vi "SR201_set_state2.vi"(8 "error in":errorcluster, 9 "state_ch2":bool, 10 "state_ch1":bool, 11 "conn_id_in":refnum<k5>) -> (0 "error out":errorcluster, 1 "ch2":bool, 2 "ch1":bool, 3 "conn_id_out":refnum<k5>, 4 "status":bool, 5 "string":string)   [LabVIEW 2019]
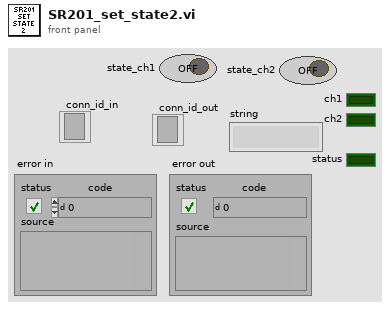
[diagram p1: front panel]
types:
  T1 = enum16{"Standard", "Buffered", "CRLF", "Immediate"}
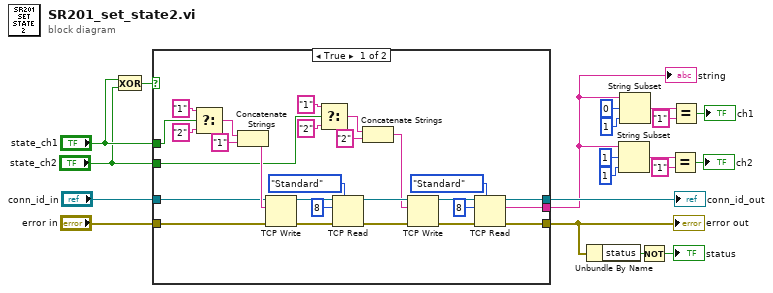
[diagram p0: block diagram]
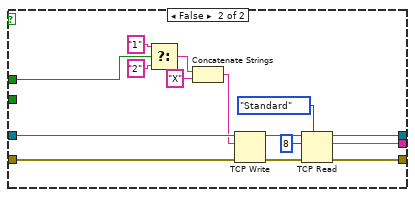
[diagram p2: hidden frame]
diagram:
  n1 = Exclusive Or(1:"state_ch2", 2:"state_ch1") -> (0:w2:bool)
  n2 = case shown="True" w2 {
    tunnel: "error in" -> [w27 w62]
    tunnel: [w39 w57] -> w19
    tunnel: "conn_id_in" -> [w28 w56]
    tunnel: [w38 w55] -> w17
    tunnel: [w37 w54] -> w4
    tunnel: "state_ch1" -> [w36 w48]
    tunnel: "state_ch2" -> [w22 _]
    frame True {
      n3 = Select(t="1", s=w36, f="2") -> (s? t:f=w41:string)
      n4 = Concatenate Strings(w41, "1" ("string")) -> (w29:string)
      n5 = TCP Write(connection ID=w28, data in=w29, error in (no error)=w27) -> (connection ID out=w34:refnum<k5>, error out=w35:errorcluster)  [unwired: 1 in, 1 out]
      n6 = Select(t="1", s=w22, f="2") -> (s? t:f=w24:string)
      n7 = TCP Read(connection ID=w34, bytes to read=8, error in (no error)=w35, 7:T1."Standard" ("mode (standard)")) -> (connection ID out=w30:refnum<k5>, error out=w31:errorcluster)  [unwired: 1 in, 1 out]
      n8 = Concatenate Strings(w24, "2" ("string")) -> (w21:string)
      n9 = TCP Write(connection ID=w30, data in=w21, error in (no error)=w31) -> (connection ID out=w46:refnum<k5>, error out=w47:errorcluster)  [unwired: 1 in, 1 out]
      n10 = TCP Read(connection ID=w46, bytes to read=8, error in (no error)=w47, 7:T1."Standard" ("mode (standard)")) -> (connection ID out=w39:refnum<k5>, data out=w37:string, error out=w38:errorcluster)  [unwired: 1 in]
    }
    frame False {
      n11 = Select(t="1", s=w48, f="2") -> (s? t:f=w51:string)
      n12 = Concatenate Strings(w51, "X" ("string")) -> (w50:string)
      n13 = TCP Write(connection ID=w56, data in=w50, error in (no error)=w62) -> (connection ID out=w60:refnum<k5>, error out=w61:errorcluster)  [unwired: 1 in, 1 out]
      n14 = TCP Read(connection ID=w60, bytes to read=8, error in (no error)=w61, 7:T1."Standard" ("mode (standard)")) -> (connection ID out=w57:refnum<k5>, data out=w54:string, error out=w55:errorcluster)  [unwired: 1 in]
    }
  }
  "error out" <- w17
  "string" <- w4
  "conn_id_out" <- w19
  n15 = Unbundle By Name(w17) -> ("status"=w16:bool)
  n16 = String Subset(string=w4, offset (0)=1, length (rest)=1 ("length (rest)")) -> (substring=w7:string)
  n17 = String Subset(string=w4, offset (0)=0, length (rest)=1 ("length (rest)")) -> (substring=w12:string)
  n18 = Not(x=w16) -> (.not. x?=→"status":bool)
  n19 = Equal?(x=w7, y="1") -> (x = y?=→"ch2":bool)
  n20 = Equal?(x=w12, y="1") -> (x = y?=→"ch1":bool)
